vi "V7310.Check.vi"(10 "Data in":string) -> (1 "Error Level":T1, 2 "Data out":string)   [LabVIEW 2016]
uses:
  V7310.ErrorLevels.ctl
panel:
  out "status":string
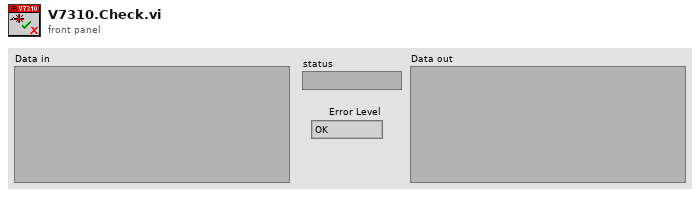
[diagram p1: front panel]
types:
  T1 = typedef "V7310.ErrorLevels.ctl" = enum16{"OK", "Warning", "Error"}
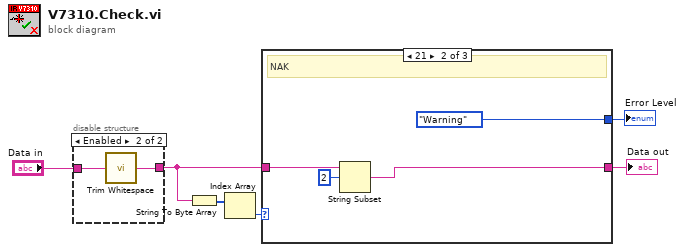
[diagram p0: block diagram]
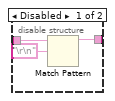
[diagram p2: hidden frame]
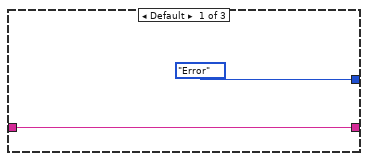
[diagram p3: hidden frame]
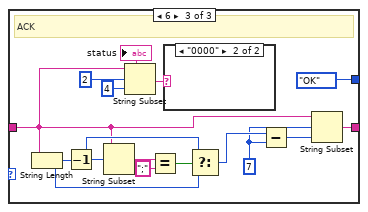
[diagram p4: hidden frame]
diagram:
  n1 = disable-structure shown="Enabled" {
    disable-tunnel: "Data in" -> [w8 w11]
    disable-tunnel: [w7 w10] -> w1
    frame Disabled {
      n2 = Match Pattern(string=w8, regular expression="\r\n") -> (before substring=w7:string)  [unwired: 1 in, 3 out]
    }
    frame Enabled {
      n3 = call <vilib>:"Trim Whitespace.vi"("string"=w11) -> ("trimmed string"=w10:string)  [unwired: 1 in]
    }
  }
  n4 = String To Byte Array(string=w1) -> (unsigned byte array=w4:u8[])
  n5 = Index Array(array=w4) -> (element=w3:u8)  [unwired: 1 in]
  n6 = case shown="21" w3 {
    tunnel: [V7310.ErrorLevels."Error" ("Error Level") V7310.ErrorLevels."Warning" ("Error Level") V7310.ErrorLevels."OK" ("Error Level")] -> w6
    tunnel: w1 -> [w12 w15 w20]
    tunnel: [w12 w14 w31] -> w2
    frame Default {
    }
    frame 21 {
      # "NAK"
      n7 = String Subset(string=w15, offset (0)=2) -> (substring=w14:string)  [unwired: 1 in]
    }
    frame 6 {
      w23 = 7 ("offset (0)")
      # "ACK"
      n8 = String Length(string=w20) -> (length=w25:i32)
      n9 = Decrement(x=w25) -> (x-1=w26:i32)
      n10 = String Subset(string=w20, offset (0)=w26) -> (substring=w30:string)  [unwired: 1 in]
      n11 = String Subset(string=w20, offset (0)=2, length (rest)=4 ("length (rest)")) -> (substring=w19:string)
      "status" <- w19
      n12 = Equal?(x=w30, y=";") -> (x = y?=w27:bool)
      n13 = case shown="\"0000\"" w19 {
        frame Default {
        }
        frame "0000" {
        }
      }
      n14 = Select(t=w26, s=w27, f=w25) -> (s? t:f=w24:i32)
      n15 = Subtract(x=w24, y=w23) -> (x-y=w28:i32)
      n16 = String Subset(string=w20, offset (0)=w23, length (rest)=w28) -> (substring=w31:string)
    }
  }
  "Data out" <- w2
  "Error Level" <- w6
